vi "AB_Engine_Package_App.vi"(5 "processed_sourceItems":T1, 7 "application package path":path, 8 "error in (no error)":errorcluster, 10 "destinations":refnum<class "AB_Destination.lvclass">[](array[class]), 11 "internal directory":path) -> (0 "error out":errorcluster, 2 "support dir":path, 3 "dup internal directory":path)   [LabVIEW 2020]
uses:
  <vilib>/AppBuilder/AB_Classes/Destination/AB_Destination.lvclass
  <vilib>/AppBuilder/AB_Classes/Source/AB_Source_Processed_Info.ctl
  <vilib>/AppBuilder/AB_CopyFiles_Data.ctl
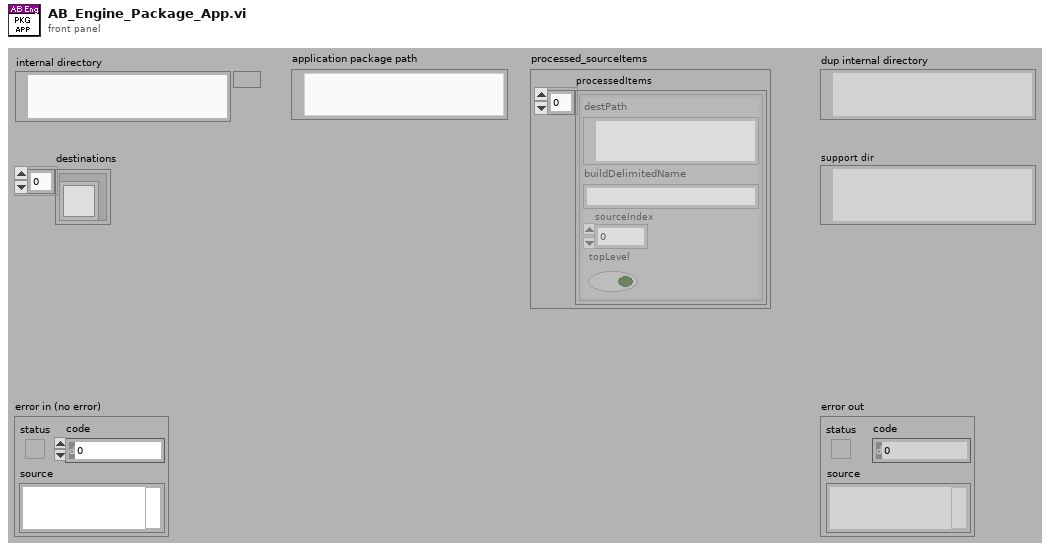
[diagram p1: front panel]
types:
  T1 = typedef "AB_CopyFiles_Data.ctl" = cluster{"processedItems":T2[]}
  T2 = typedef "AB_Source_Processed_Info.ctl" = cluster{"destPath":path, "buildDelimitedName":string, "sourceIndex":i32, "topLevel":bool}
  T3 = enum32{"invalid OS target", "Mac OS", "Windows 3.1", "Windows 95/NT", "Solaris 1", "Solaris 2", "HP-UX", "PowerMAX", "Linux", "Irix", "Rhapsody", "BeOS", "AIX", "OSF1", "VxWorks", "PharLap", "Carbon", "RTX", "Windows x64", "Linux x64", "Mac OS X x64"}
  T4 = typedef "AB_Destination.ctl" = cluster{"destName":string, "path":path, "libraryName":string, "preserveHierarchy":bool, "eng_inBuild":bool, "eng_libraryReference":refnum<vi>, "eng_restictAddToNewLibrary":bool}
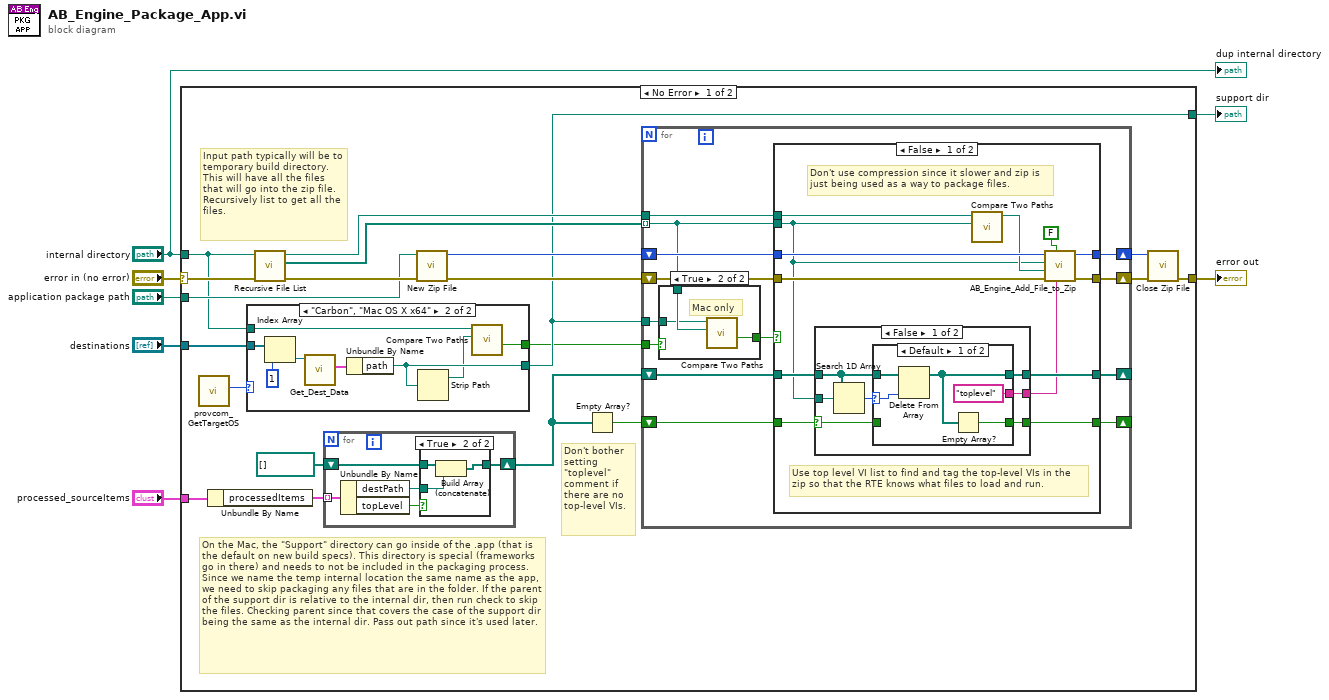
[diagram p0: block diagram]
diagram:
  n1 = case shown="No Error" "error in (no error)" {
    selector: "error in (no error)" -> [w17 w94]
    tunnel: [w27 w94] -> w7
    tunnel: "internal directory" -> [w13 _]
    tunnel: "application package path" -> [w18 _]
    tunnel: "destinations" -> [w15 _]
    tunnel: [w14 _] -> w2
    tunnel: "processed_sourceItems" -> [w10 _]
    frame No Error {
      # "On the Mac, the \"Support\" directory can go inside of the .app (that is the default on new build specs). This directory is special (frameworks go in there) and needs to not be included in the packaging process. Since we name the temp internal location the same name as the app, we need to skip packaging any files that are in the folder. If the parent of the support dir is relative to the internal dir, then run check to skip the files. Checking parent since that covers the case of the support dir being the same as the internal dir. Pass out path since it's used later."
      # "Don't bother setting \"toplevel\" comment if there are no top-level VIs."
      # "Input path typically will be to temporary build directory. This will have all the files that will go into the zip file. Recursively list to get all the files."
      n2 = call <resource>:"provcom_GetTargetOS.vi"() -> ("App.TargetOS"=w16:T3)  [unwired: 11 out]
      n3 = Unbundle By Name(w10) -> ("processedItems"=w11:T2[])
      n4 = case shown="\"Carbon\", \"Mac OS X x64\"" w16 {
        tunnel: w15 -> [_ w41]
        tunnel: [_ w40] -> w14
        tunnel: w13 -> [_ w39]
        tunnel: [_ w37] -> w12
        frame Default {
        }
        frame "Carbon", "Mac OS X x64" {
          n5 = Index Array(array=w41, index=1) -> (element=w44:refnum<class "AB_Destination.lvclass">)
          n6 = call <vilib>:"Get_Dest_Data.vi"("Class in"=w44) -> ("destName"=w43:T4)  [unwired: 1 in, 9 out]
          n7 = Unbundle By Name(w43) -> ("path"=w40:path)
          n8 = Strip Path(path=w40) -> (stripped path=w38:path)  [unwired: 1 out]
          n9 = call <vilib>:"Compare Two Paths.vi"("Path 2"=w38, "Path 1"=w39) -> ("Path 2 Relative to Path 1?"=w37:bool)  [unwired: 1 in, 8 out]
        }
      }
      n10 = call <vilib>:"Recursive File List.vi"("error in (no error)"=w17, "Folder Path"=w13) -> ("error out"=w19:errorcluster, "All Files in Dir"=w22:path[], "dup Folder Path"=w20:path)  [unwired: 1 in, 6 out]
      n11 = for {
        tunnel: w11 -> [w32] mode=indexing
        shift-right: [w29] -> w8
        shift-left: path[] [] -> [w28]
        n12 = Unbundle By Name(w32) -> ("destPath"=w30:path, "topLevel"=w31:bool)
        n13 = case shown="True" w31 {
          tunnel: w30 -> [_ w36]
          tunnel: [w33 w35] -> w29
          tunnel: w28 -> [w33 w34]
          frame False {
          }
          frame True {
            n14 = Build Array (concatenate)(w34, w36) -> (w35:path[])
          }
        }
      }
      n15 = call <vilib>:"New Zip File.vi"("error in (no error)"=w19, "target"=w18) -> ("error out"=w23:errorcluster, "zip file out"=w26:i64)  [unwired: 1 in, 3 out]
      n16 = Empty Array?(array=w8) -> (empty?=w21:bool)
      n17 = for {
        shift-right: [w56] -> w25
        shift-left: w26 -> [w57]
        shift-right: [w55] -> w24
        shift-left: w23 -> [w54]
        tunnel: w22 -> [w48] mode=indexing
        tunnel: w20 -> [w53]
        shift-right: [w52] -> _
        shift-left: w8 -> [w51]
        shift-right: [w49] -> _
        shift-left: w21 -> [w50]
        tunnel: w14 -> [w47]
        tunnel: w12 -> [w45]
        n18 = case shown="True" w45 {
          tunnel: w48 -> [_ w60]
          tunnel: w47 -> [_ w59]
          tunnel: [_ w58] -> w46
          frame False {
          }
          frame True {
            # "Mac only"
            n19 = call <vilib>:"Compare Two Paths.vi"("Path 2"=w60, "Path 1"=w59) -> ("Path 2 Relative to Path 1?"=w58:bool)  [unwired: 1 in, 8 out]
          }
        }
        n20 = case shown="False" w46 {
          tunnel: w57 -> [w73 w90]
          tunnel: [w72 w90] -> w56
          tunnel: [w71 w91] -> w55
          tunnel: w54 -> [w70 w91]
          tunnel: w53 -> [w69 _]
          tunnel: w48 -> [w61 _]
          tunnel: [w66 w92] -> w52
          tunnel: w51 -> [w64 w92]
          tunnel: w50 -> [w63 w93]
          tunnel: [w62 w93] -> w49
          frame False {
            # "Don't use compression since it slower and zip is just being used as a way to package files."
            # "Use top level VI list to find and tag the top-level VIs in the zip so that the RTE knows what files to load and run."
            n21 = case shown="False" w63 {
              selector: w63 -> [w75 w88]
              tunnel: w61 -> [w80 _]
              tunnel: [w78 w89] -> w66
              tunnel: [w77 _] -> w65
              tunnel: w64 -> [w76 w89]
              tunnel: [w74 w88] -> w62
              frame False {
                n22 = Search 1D Array(1D array=w76, element=w80) -> (index of element=w79:i32)  [unwired: 1 out]
                n23 = case shown="Default" w79 {
                  selector: w79 -> [w83 _]
                  tunnel: w76 -> [w84 w87]
                  tunnel: [w82 w87] -> w78
                  tunnel: ["toplevel" _] -> w77
                  tunnel: w75 -> [_ w86]
                  tunnel: [w81 w86] -> w74
                  frame Default {
                    n24 = Delete From Array(array=w84, index=w83) -> (array with subset deleted=w82:path[])  [unwired: 1 in, 1 out]
                    n25 = Empty Array?(array=w82) -> (empty?=w81:bool)
                  }
                  frame -1 {
                  }
                }
              }
              frame True {
              }
            }
            n26 = call <vilib>:"Compare Two Paths.vi"("Path 2"=w61, "Path 1"=w69) -> ("Relative Path from 1 to 2"=w68:path)  [unwired: 1 in, 8 out]
            n27 = call <vilib>:"AB_Engine_Add_File_to_Zip.vi"("Comment"=w65, "Compress (T)"=FALSE, "error in (no error)"=w70, "destination path in zip"=w68, "source file path"=w61, "zip file in"=w73) -> ("error out"=w71:errorcluster, "zip file out"=w72:i64)  [unwired: 4 out]
          }
          frame True {
          }
        }
      }
      n28 = call <vilib>:"Close Zip File.vi"("error in (no error)"=w24, "zip file in"=w25) -> ("error out"=w27:errorcluster)  [unwired: 1 in, 4 out]
    }
    frame Error {
    }
  }
  "error out" <- w7
  "support dir" <- w2
  "dup internal directory" <- "internal directory"
